vi "soilwave.vi"() -> ()   [LabVIEW 2012]
panel:
  in  "Time":dbl(slide)=113.20754716981132 scale=0.0..144.0
  out "XY Graph":cluster{dbl[], i32[]}(graph)={[16.305261922200526, 16.55591917620975, 16.789163728954794, 17.005603081559176, 17.205838830662426, 17.3904659526893, 17.56007214168079, 17.71523719872029, 17.856532471013157, 17.98452033870318, 18.099753747538102, 18.20277578552527, 18.294119301750342, 18.374306565563835, 18.443848964374805, 18.503246738325245, 18.55298875015536, 18.593552288606094, 18.62540290374348, 18.648994272627007, 18.664768093783586, 18.67315400898738, 18.674569550885774, 18.66942011505128, 18.65809895507943, 18.640987199392608, 18.61845388845005, 18.59085603110419, 18.558538678883632, 18.52183501702249, 18.481066471095772, 18.436542828159293, 18.38856237133174, 18.33741202679479, 18.283367522225397, 18.22669355571163, 18.167643974240764, 18.106461960884467, 18.04338022984206, 17.97862122853788, 17.912397346003416, 17.844911126808945, 17.776355489842455, 17.70691395126626, 17.636760851013584, 17.566061582218385, 17.494972823002, 17.423642770069893, 17.35221137360043, 17.28081057293577, 17.20956453261212, 17.138589878293168, 17.067995932196112, 16.997884947624712, 16.928352342247884, 16.859486929785714, 16.791371149787373, 16.724081295207295, 16.657687737506933, 16.592255149029885, 16.527842722417574, 16.464504386851683, 16.402289020927498, 16.341240661979867, 16.28139871170005, 16.22279813789778, 16.165469672278252, 16.10944000411827, 16.054731969739937, 16.001364737693528, 15.949353989573975, 15.898712096407497, 15.849448290556463, 15.801568833101499, 15.755077176670202, 15.70997412369173, 15.666257980065705, 15.623924704242762, 15.58296805172219, 15.54337971498001, 15.505149458847995, 15.468265251371069, 15.432713390176787, 15.398478624396663, 15.365544272184504, 15.33389233388213, 15.303503600887556, 15.27435776028506, 15.246433495300574, 15.219708581649474, 15.194159979847207, 15.169763923556102, 15.146496004044542, 15.124331250836946, 15.103244208635225, 15.0832090105942, 15.064199448035072, 15.046189036682417, 15.029151079511275, 15.013058726291868], [0, 1, 2, 3, 4, 5, 6, 7, 8, 9, 10, 11, 12, 13, 14, 15, 16, 17, 18, 19, 20, 21, 22, 23, 24, 25, 26, 27, 28, 29, 30, 31, 32, 33, 34, 35, 36, 37, 38, 39, 40, 41, 42, 43, 44, 45, 46, 47, 48, 49, 50, 51, 52, 53, 54, 55, 56, 57, 58, 59, 60, 61, 62, 63, 64, 65, 66, 67, 68, 69, 70, 71, 72, 73, 74, 75, 76, 77, 78, 79, 80, 81, 82, 83, 84, 85, 86, 87, 88, 89, 90, 91, 92, 93, 94, 95, 96, 97, 98, 99]}
  in  "Boolean":bool
  in  "Depth (m)":dbl(slide)=0.3563829787234043
  in  "Thermal diffusivity (m2 s-1)":dbl(slide)=4e-06 scale=1e-08..1e-05
  out "Intensity Graph":dbl[][](graph)
  out "Waveform Graph":dbl[][](graph)=[[5.603073792140918, 5.46283049251773, 5.340741737109317, 5.237039928800666, 5.1519224698779205, 5.085551386261896, 5.038053019082545, 5.009517784181423, 5.0, 5.009517784181423, 5.038053019082545, 5.085551386261894, 5.151922469877919, 5.237039928800666, 5.340741737109315, 5.46283049251773, 5.603073792140915, 5.76120467488713, 5.936922129633498, 6.129891668217784, 6.3397459621556145, 6.566085541871143, 6.808479557110083, 7.066466597087649, 7.339555568810219, 7.627226631898758, 7.928932188134523, 8.244097923843395, 8.572123903134603, 8.91238570991279, 9.264235636489534, 9.627003916531757, 9.999999999999996, 10.382513867649656, 10.773817382593, 11.173165676349097, 11.579798566743307, 11.99294200495727, 12.411809548974793, 12.83560386061897, 13.263518223330696, 13.694738077799483, 14.128442572523417, 14.563806126346638, 14.999999999999998, 15.436193873653357, 15.871557427476578, 16.30526192220051, 16.7364817766693, 17.164396139381026, 17.588190451025202, 18.007057995042725, 18.42020143325668, 18.826834323650893, 19.226182617406987, 19.617486132350333, 20.0, 20.372996083468237, 20.735764363510462, 21.087614290087206, 21.42787609686539, 21.7559020761566, 22.071067811865476, 22.37277336810124, 22.660444431189777, 22.93353340291235, 23.191520442889914, 23.433914458128854, 23.660254037844382, 23.870108331782212, 24.0630778703665, 24.238795325112864, 24.39692620785908, 24.537169507482268, 24.65925826289068, 24.762960071199334, 24.84807753012208, 24.914448613738102, 24.961946980917453, 24.990482215818577, 25.0, 24.990482215818577, 24.961946980917453, 24.914448613738106, 24.848077530122083, 24.76296007119933, 24.659258262890685, 24.537169507482268, 24.39692620785909, 24.238795325112868, 24.063077870366502, 23.87010833178222, 23.66025403784439, 23.433914458128857, 23.191520442889924, 22.933533402912353, 22.660444431189788, 22.372773368101242, 22.071067811865483, 21.755902076156605, 21.427876096865404, 21.08761429008721, 20.73576436351046, 20.372996083468244, 20.0, 19.617486132350344, 19.226182617406995, 18.826834323650907, 18.420201433256686, 18.00705799504274, 17.58819045102521, 17.16439613938104, 16.736481776669304, 16.305261922200526, 15.871557427476585, 15.436193873653371, 15.000000000000004, 14.563806126346654, 14.128442572523422, 13.69473807779948, 13.263518223330703, 12.835603860618969, 12.411809548974798, 11.992942004957268, 11.579798566743321, 11.173165676349102, 10.773817382593013, 10.38251386764966, 10.000000000000007, 9.627003916531763, 9.264235636489548, 8.912385709912796, 8.572123903134615, 8.2440979238434, 7.928932188134534, 7.627226631898763, 7.339555568810229, 7.0664665970876515, 6.808479557110081, 6.566085541871146, 6.339745962155613, 6.129891668217786, 5.9369221296334995, 5.761204674887136], [14.499055326278818, 14.352196664427758, 14.206571133044699, 14.062455938605439, 13.920125412573562, 13.779850489194912, 13.641898189758844, 13.50653111430803, 13.374006941764353, 13.244577939422435, 13.11849048274449, 12.995984586370653, 12.877293447237449, 12.762643000674181, 12.65225149032219, 12.546329052695672, 12.445077317174889, 12.348689022193174, 12.257347648348382, 12.171227069137124, 12.090491219976709, 12.015293786144738, 11.94577791023045, 11.882075919654676, 11.824309074777057, 11.772587338070075, 11.72700916479922, 11.687661315607809, 11.654618691363158, 11.627944190578546, 11.607688589682287, 11.593890446361947, 11.586576026167567, 11.585759252513714, 11.591441680175459, 11.60361249232878, 11.622248521141, 11.647314291872073, 11.678762090402765, 11.716532054061199, 11.760552285574844, 11.810738989931071, 11.866996633885709, 11.929218127816018, 11.997285029571858, 12.071067769937073, 12.150425899271836, 12.235208354866542, 12.325253748498241, 12.420390673642316, 12.520438031754518, 12.625205377002368, 12.734493278789593, 12.848093701383632, 12.965790399923442, 13.087359332053916, 13.212569084403215, 13.34118131309128, 13.472951197430971, 13.607627905958127, 13.744955073903554, 13.88467129119789, 14.026510600080577, 14.170203001365525, 14.315474968399958, 14.462049967737894, 14.60964898553733, 14.75799105867889, 14.906793809595149, 15.055773983792331, 15.204647989041385, 15.353132435211862, 15.500944673721184, 15.647803335572236, 15.7934288669553, 15.937544061394563, 16.079874587426435, 16.22014951080509, 16.358101810241156, 16.49346888569197, 16.625993058235643, 16.75542206057757, 16.88150951725551, 17.004015413629347, 17.12270655276255, 17.23735699932582, 17.347748509677807, 17.453670947304328, 17.55492268282511, 17.651310977806826, 17.742652351651618, 17.828772930862876, 17.909508780023287, 17.98470621385526, 18.054222089769546, 18.117924080345325, 18.17569092522294, 18.227412661929925, 18.27299083520078, 18.31233868439219, 18.34538130863684, 18.372055809421454, 18.392311410317713, 18.406109553638053, 18.413423973832433, 18.414240747486286, 18.408558319824543, 18.39638750767122, 18.377751478859, 18.35268570812793, 18.321237909597237, 18.283467945938803, 18.239447714425157, 18.189261010068932, 18.13300336611429, 18.070781872183986, 18.002714970428144, 17.92893223006293, 17.849574100728166, 17.764791645133457, 17.67474625150176, 17.579609326357684, 17.479561968245484, 17.374794622997634, 17.265506721210407, 17.151906298616368, 17.034209600076558, 16.912640667946086, 16.78743091559679, 16.65881868690872, 16.527048802569034, 16.392372094041875, 16.255044926096453, 16.11532870880211, 15.97348939991943, 15.829796998634476, 15.68452503160005, 15.537950032262106, 15.390351014462672, 15.242008941321112, 15.093206190404851, 14.944226016207669, 14.795352010958615, 14.646867564788138]]
  in  "Surface T-wave amplitude (K)":dbl(slide)=10.0 scale=0.0..10.0
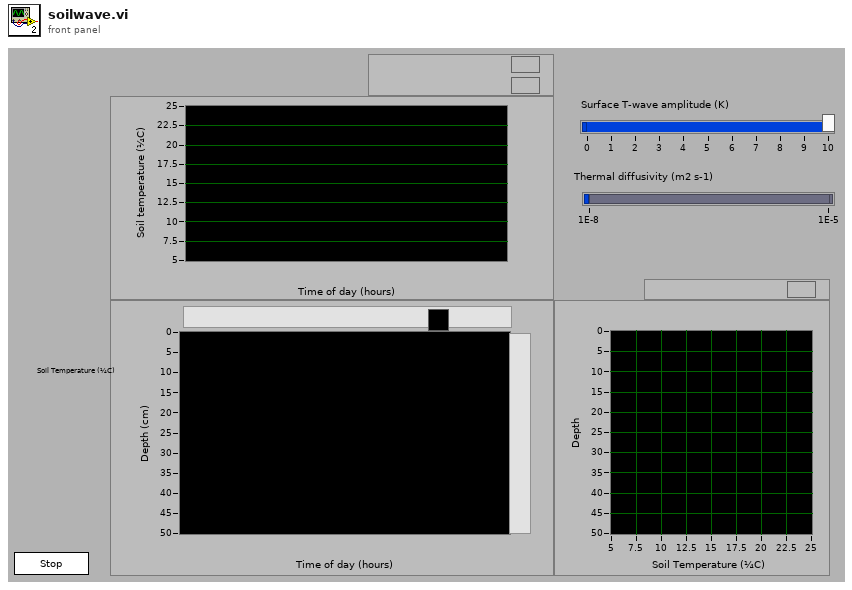
[diagram p1: front panel]
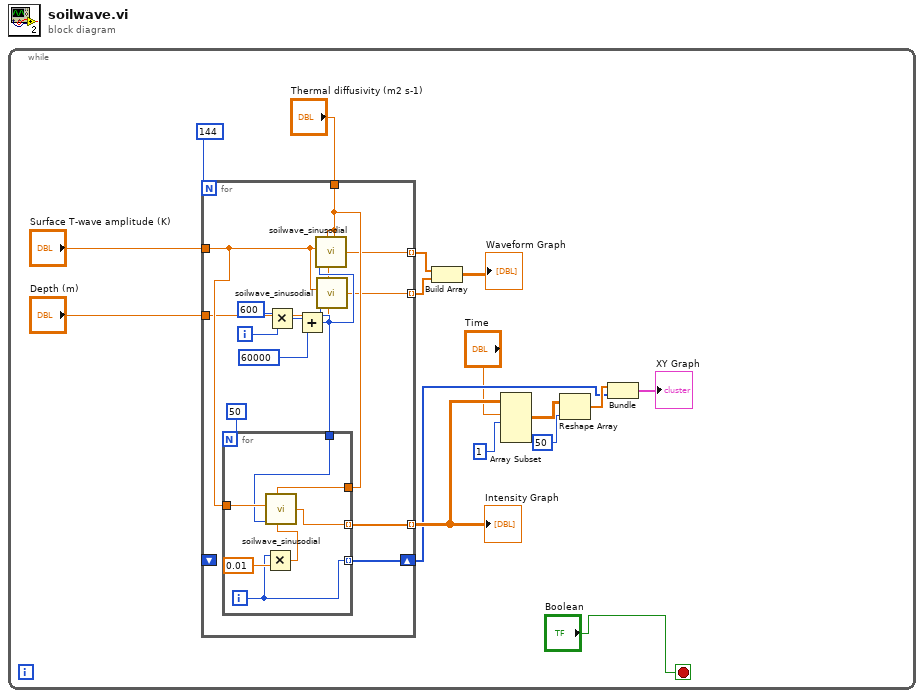
[diagram p0: block diagram]
diagram:
  n1 = while {
    stop <- "Boolean" stop-if-true
    n2 = for {
      N: 144 -> [_]
      tunnel: "Surface T-wave amplitude (K)" -> [w21]
      tunnel: [w25] -> w9 mode=indexing
      tunnel: "Thermal diffusivity (m2 s-1)" -> [w22]
      tunnel: "Depth (m)" -> [w20]
      tunnel: [w19] -> w12 mode=indexing
      tunnel: [w18] -> w11 mode=indexing
      shift-right: [w17] -> w4
      shift-left: _ -> [_]
      i -> [w29]
      n3 = Multiply(x=600, y=w29) -> (x*y=w27:i32)
      n4 = Add(x=w27, y=60000) -> (x+y=w23:i32)
      n5 = for {
        N: 50 -> [_]
        tunnel: [w36] -> w25 mode=indexing
        tunnel: w21 -> [w35]
        tunnel: w23 -> [w34]
        tunnel: w22 -> [w32]
        tunnel: [w30] -> w17 mode=indexing
        i -> [w30]
        n6 = Multiply(x=w30, y=0.01) -> (x*y=w31:dbl)
        n7 = call "soilwave_sinusodial.vi"("Depth (m)"=w31, "Thermal diffusivity (m2 s-1)"=w32, "Time (s)"=w34, "Surface temperature amplitude (K)"=w35) -> ("Soil temperature (z,t) (¼C)"=w36:dbl)  [unwired: 2 in]
      }
      n8 = call "soilwave_sinusodial.vi"("Thermal diffusivity (m2 s-1)"=w22, "Time (s)"=w23, "Surface temperature amplitude (K)"=w21) -> ("Soil temperature (z,t) (¼C)"=w19:dbl)  [unwired: 3 in]
      n9 = call "soilwave_sinusodial.vi"("Depth (m)"=w20, "Thermal diffusivity (m2 s-1)"=w22, "Time (s)"=w23, "Surface temperature amplitude (K)"=w21) -> ("Soil temperature (z,t) (¼C)"=w18:dbl)  [unwired: 2 in]
    }
    "Intensity Graph" <- w9
    n10 = Build Array(w12, w11) -> (→"Waveform Graph":dbl[][])
    n11 = Array Subset(array=w9, index (row)="Time", length (row)=1 ("length")) -> (w7:dbl[][])  [unwired: 2 in]
    n12 = Reshape Array(w7, 50 ("dimension size")) -> (w5:dbl[])
    n13 = Bundle(w5, w4) -> (→"XY Graph":cluster{dbl[], i32[]})  [unwired: 1 in]
  }
